vi "Store Step Result.vi"(8 "error in (no error)":errorcluster, 10 "SequenceContext Ref":refnum<k7>, 11 "Execution in":refnum<class "Execution.lvclass">) -> (0 "error out":errorcluster, 3 "Execution out":refnum<class "Execution.lvclass">)   [LabVIEW 2020, in "TSnax.lvlib" / "Execution.lvclass"]
uses:
  Execution.lvclass
  Execution.lvclass/Execution.ctl
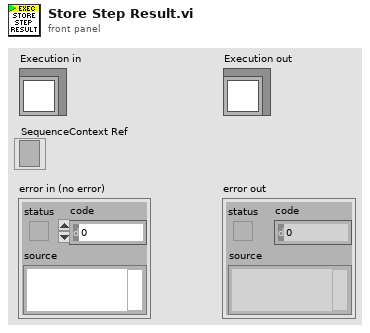
[diagram p1: front panel]
types:
  T1 = typedef "TSnax.lvlib/Execution.lvclass/Step Results.ctl" = cluster{"Map":map{string, string}}
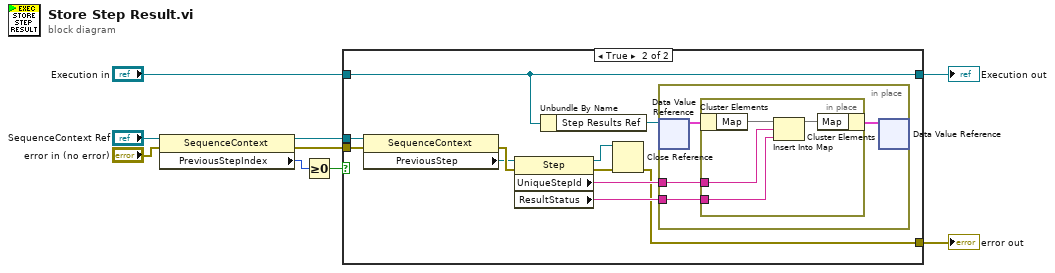
[diagram p0: block diagram]
diagram:
  n1 = property class="SequenceContext"(reference="SequenceContext Ref", error in="error in (no error)") -> (reference out=w5:refnum<k7>, error out=w4:errorcluster, "PreviousStepIndex"=w8:i32)
  n2 = Greater Or Equal To 0?(x=w8) -> (x >= 0?=w6:bool)
  n3 = case shown="True" w6 {
    tunnel: w5 -> [_ w21]
    tunnel: w4 -> [w11 w20]
    tunnel: "Execution in" -> [w10 w12]
    tunnel: [w11 w13] -> w2
    tunnel: [w10 w12] -> w1
    frame False {
    }
    frame True {
      n4 = property class="SequenceContext"(reference=w21, error in=w20) -> (error out=w22:errorcluster, "PreviousStep"=w19:refnum<k7>)  [unwired: 1 out]
      n5 = property class="Step"(reference=w19, error in=w22) -> (reference out=w17:refnum<k7>, error out=w18:errorcluster, "UniqueStepId"=w15:string, "ResultStatus"=w14:string)
      n6 = Unbundle By Name(w12) -> ("Step Results Ref"=w16:refnum<data-value>)
      n7 = Close Reference(reference=w17, error in (no error)=w18) -> (error out=w13:errorcluster)
      n8 = in-place {
        in-place-border: w15 -> [w24]
        in-place-border: w14 -> [w23]
        n9 = in-place-dvr #1(w16) -> (w26:T1)  [unwired: 1 out]
        n10 = in-place {
          in-place-border: w24 -> [w29]
          in-place-border: w23 -> [w28]
          n11 = in-place-cluster #2(w26) -> ("Map"=w30:map{string, string})
          n12 = Insert Into Map(map in=w30, key=w29, value=w28) -> (map out=w27:map{string, string})  [unwired: 2 out]
          n13 = in-place-cluster #2("Map"=w27) -> (w25:T1)
        }
        n14 = in-place-dvr #1(w25) -> ()  [unwired: 2 out]
      }
    }
  }
  "error out" <- w2
  "Execution out" <- w1
